vi "field_to_voltage_convert.vi"(1 "Start H Field (Oe)":dbl) -> (0 "Numeric":dbl)   [LabVIEW 2017]
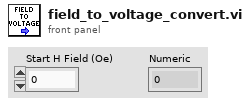
[diagram p1: front panel]
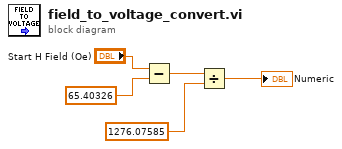
[diagram p0: block diagram]
diagram:
  n1 = Subtract(x="Start H Field (Oe)", y=65.40326) -> (x-y=w3:dbl)
  n2 = Divide(x=w3, y=1276.07585) -> (x/y=→"Numeric":dbl)
